vi "tsfifo_receive_can_message_win32.vi"(8 "错误输入（无错误）":errorcluster, 9 "AOnlyRx":u8, 10 "AAppChannel输入":i32) -> (0 "错误输出":errorcluster, 1 "tsapp_receive_can_message":bool, 4 "Receive message":T1)   [LabVIEW 2016]
uses:
  MessageInfo.ctl
  SendMsgInfo.ctl
  TSMaster.dll
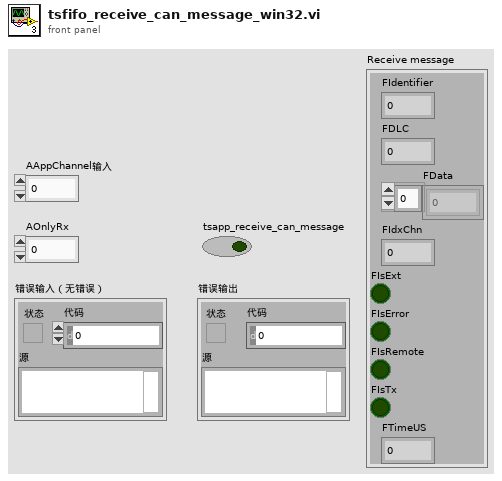
[diagram p1: front panel]
types:
  T1 = typedef "MessageInfo.ctl" = cluster{"FIdentifier":i32, "FDLC":u8, "FData":u8[], "FIdxChn":u8, "FIsExt":bool, "FIsError":bool, "FIsRemote":bool, "FIsTx":bool, "FTimeUS":u64}
  T2 = typedef "SendMsgInfo.ctl" = cluster{"FIdxChn":u8, "FProperties":u8, "FDLC":u8, "FReserved":u8, "FIdentifier":i32, "FTimeUS":u64, "Data0":u8, "Data1":u8, "Data2":u8, "Data3":u8, "Data4":u8, "Data5":u8, "Data6":u8, "Data7":u8}
  T3 = typedef "TCANProperty.ctl" = cluster{"istx":bool, "remoteframe":bool, "extframe":bool, "tbd1":bool, "tbd2":bool, "tbd3":bool, "tbd4":bool, "iserrorframe":bool}
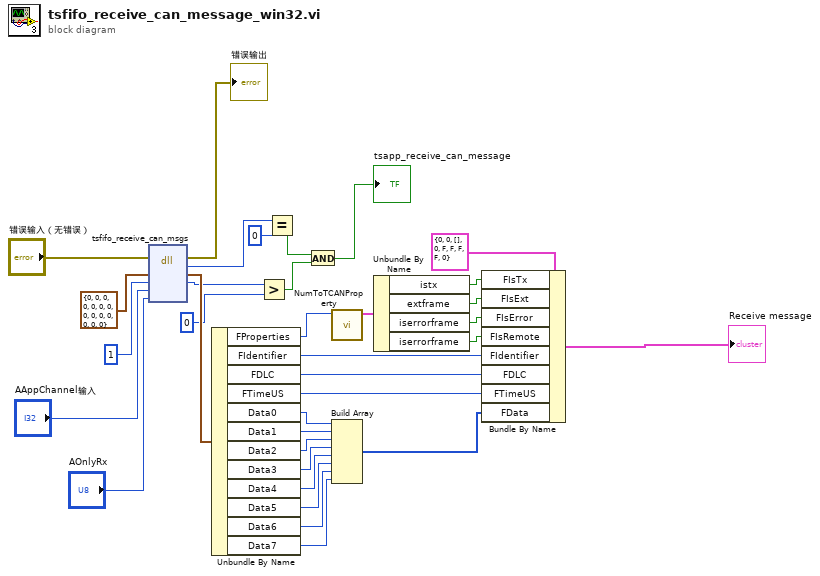
[diagram p0: block diagram]
diagram:
  n1 = dll-call lib="C:/Users/Eric/Desktop/LabVIEW/TSMasterAPI/Win32/TSMaster_LV2010_Release/TSMaster.dll" fn="tsfifo_receive_can_msgs"(error in="错误输入（无错误）", "ACANBuffers"=T2 {"FIdxChn"=0, "FProperties"=0, "FDLC"=0, "FReserved"=0, "FIdentifier"=0, "FTimeUS"=0, "Data0"=0, "Data1"=0, "Data2"=0, "Data3"=0, "Data4"=0, "Data5"=0, "Data6"=0, "Data7"=0} ("SendMsgInfo"), "ACANBufferSize"=1, "AChn"="AAppChannel输入", "ARxTx"="AOnlyRx") -> (error out=→"错误输出":errorcluster, "tsapp_receive_can_msgs"=w5:i32, "ACANBuffers"=w27:T2, "ACANBufferSize"=w7:i32)  [unwired: 4 in, 1 out]
  n2 = Unbundle By Name(w27) -> ("FProperties"=w26:u8, "FIdentifier"=w20:i32, "FDLC"=w19:u8, "FTimeUS"=w18:u64, "Data0"=w17:u8, "Data1"=w16:u8, "Data2"=w15:u8, "Data3"=w14:u8, "Data4"=w13:u8, "Data5"=w12:u8, "Data6"=w11:u8, "Data7"=w10:u8)
  n3 = Greater?(x=w7, y=0) -> (0:w1:bool)
  n4 = Equal?(x=w5, y=0) -> (x = y?=w3:bool)
  n5 = And(x=w3, y=w1) -> (x .and. y?=→"tsapp_receive_can_message":bool)
  n6 = call "NumToTCANProperty.vi"("TCANPropertyNum"=w26) -> ("TCANProperty"=w25:T3)  [unwired: 10 in]
  n7 = Build Array(w17, w16, w15, w14, w13, w12, w11, w10) -> (w9:u8[])
  n8 = Unbundle By Name(w25) -> ("istx"=w24:bool, "extframe"=w23:bool, "iserrorframe"=w22:bool, "iserrorframe"=w21:bool)
  n9 = Bundle By Name(cluster=T1 {"FIdentifier"=0, "FDLC"=0, "FData"=[], "FIdxChn"=0, "FIsExt"=FALSE, "FIsError"=FALSE, "FIsRemote"=FALSE, "FIsTx"=FALSE, "FTimeUS"=0} ("Receive message"), "FIsTx"=w24, "FIsExt"=w23, "FIsError"=w22, "FIsRemote"=w21, "FIdentifier"=w20, "FDLC"=w19, "FTimeUS"=w18, "FData"=w9) -> (→"Receive message":T1)
